vi "Handle.vi"(10 "log record":T1 {"timestamp" format="%<%x %.3X>T"}, 11 "logger in":refnum<class "Logger.lvclass">) -> (3 "logger out":refnum<class "Logger.lvclass">)   [LabVIEW 2018, in "GLog.lvlib" / "Logger.lvclass"]
uses:
  Logger.lvclass
  Log Record.ctl
  Internal Log Levels.ctl
  Logger.lvclass/Logger.ctl
  Failure Popup.vi
  <vilib>/ErrorRing/Error Ring.xnode
  extension/formatting_handler_interface/Formatting Handler.lvclass
  GLog.lvlib
panel:
  # "Connector Pane"
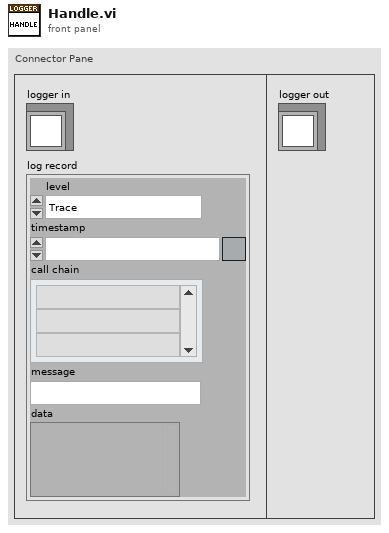
[diagram p1: front panel]
types:
  T1 = typedef "GLog.lvlib/Log Record.ctl" = cluster{"level":T2, "timestamp":timestamp, "call chain":string[], "message":string, "data":variant}
  T2 = typedef "GLog.lvlib/Internal Log Levels.ctl" = enum16{"Trace", "Debug", "Info", "Warning", "Error", "Critical", "Internal"}
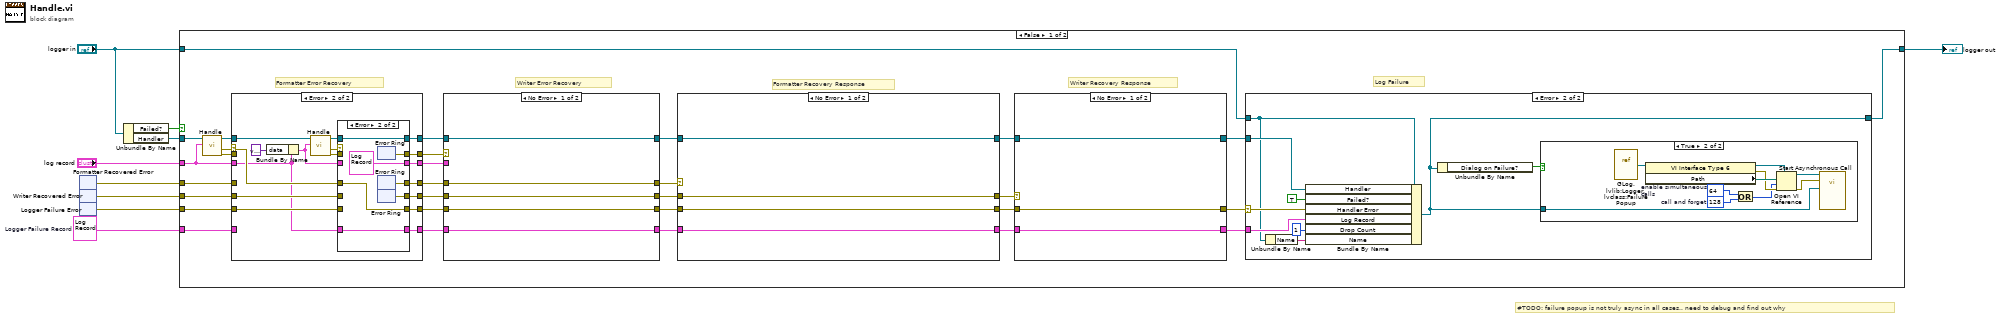
[diagram p0: block diagram]
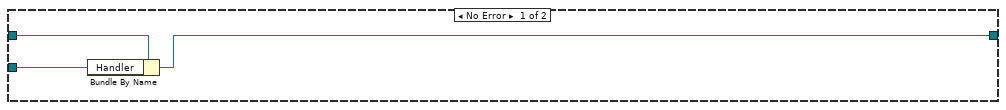
[diagram p2: hidden frame]
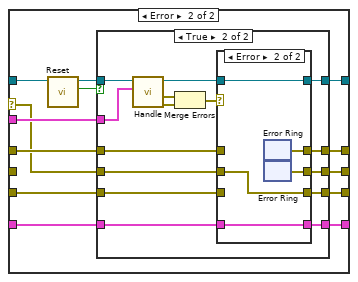
[diagram p6: hidden frame]
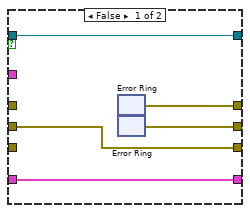
[diagram p7: hidden frame]
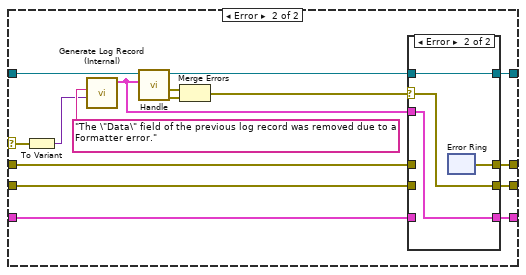
[diagram p9: hidden frame]
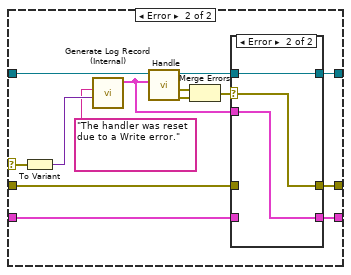
[diagram p11: hidden frame]
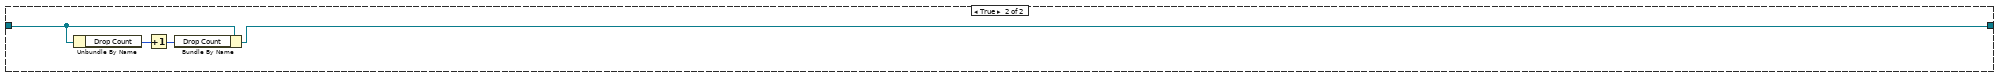
[diagram p13: hidden frame]
diagram:
  w9 = T1 {"level"=enum."Trace", "timestamp"=timestamp(0 s since 1904-01-01), "call chain"=[], "message"="", "data"=variant}  # Logger Failure Record
  # "#TODO: failure popup is not truly async in all cases.. need to debug and find out why"
  n1 = xnode "Formatter Recovered Error"() -> ("error out"=w6:errorcluster)
  n2 = xnode "Writer Recovered Error"() -> ("error out"=w7:errorcluster)
  n3 = xnode "Logger Failure Error"() -> ("error out"=w8:errorcluster)
  n4 = Unbundle By Name("logger in") -> ("Failed?"=w1:bool, "Handler"=w5:refnum<class "Formatting Handler.lvclass">)
  n5 = case shown="False" w1 {
    tunnel: w9 -> [w38 _]
    tunnel: w8 -> [w33 _]
    tunnel: w7 -> [w32 _]
    tunnel: w6 -> [w30 _]
    tunnel: w5 -> [w15 _]
    tunnel: "log record" -> [w13 _]
    tunnel: "logger in" -> [w11 w206]
    tunnel: [w10 w205] -> w2
    frame False {
      # "Log Failure"
      # "Writer Recovery Response"
      # "Formatter Recovery Response"
      # "Writer Error Recovery"
      # "Formatter Error Recovery"
      n6 = call-dynamic "Handle.vi"("log record"=w13, "handler in"=w15) -> ("writer error"=w16:errorcluster, "formatter error"=w12:errorcluster, "handler out"=w14:refnum<class "Formatting Handler.lvclass">)  [unwired: 7 in]
      n7 = case shown="Error" w12 {
        selector: w12 -> [_ w70]
        tunnel: w13 -> [w62 w68]
        tunnel: w14 -> [w63 w83]
        tunnel: w16 -> [w67 _]
        tunnel: [w67 w80] -> w17
        tunnel: [w66 w79] -> w18
        tunnel: [w64 w77] -> w19
        tunnel: w30 -> [w66 _]
        tunnel: w33 -> [w64 w78]
        tunnel: [w65 w76] -> w24
        tunnel: w32 -> [w65 w75]
        tunnel: [w63 w74] -> w27
        tunnel: [w62 w71] -> w28
        tunnel: [w62 w69] -> w37
        tunnel: w38 -> [_ _]
        frame No Error {
        }
        frame Error {
          n8 = Bundle By Name(cluster=w68, "data"=variant) -> (w72:T1)
          n9 = call-dynamic "Handle.vi"("log record"=w72, "handler in"=w83) -> ("writer error"=w81:errorcluster, "formatter error"=w82:errorcluster, "handler out"=w73:refnum<class "Formatting Handler.lvclass">)  [unwired: 7 in]
          n10 = case shown="Error" w82 {
            tunnel: w81 -> [w90 _]
            tunnel: [w90 w97] -> w80
            tunnel: [w86 w94] -> w79
            tunnel: [w89 w92] -> w77
            tunnel: w70 -> [w86 w92]
            tunnel: w78 -> [w89 _]
            tunnel: [w88 w93] -> w76
            tunnel: w75 -> [w88 _]
            tunnel: [w87 w96] -> w74
            tunnel: w73 -> [w87 w96]
            tunnel: [w85 T1 {"level"=enum."Trace", "timestamp"=timestamp(0 s since 1904-01-01), "call chain"=[], "message"="", "data"=variant} ("log record")] -> w71
            tunnel: w72 -> [w85 _]
            tunnel: [w85 w91] -> w69
            tunnel: w68 -> [_ w91]
            frame No Error {
            }
            frame Error {
              n11 = xnode "Error Ring"() -> ("error out"=w97:errorcluster)
              n12 = xnode "Error Ring"() -> ("error out"=w94:errorcluster)
              n13 = xnode "Error Ring"() -> ("error out"=w93:errorcluster)
            }
          }
        }
      }
      n14 = case shown="No Error" w17 {
        selector: w17 -> [_ w108]
        tunnel: w18 -> [w105 w113]
        tunnel: w19 -> [w104 w111]
        tunnel: [w105 w114] -> w20
        tunnel: [w104 w109] -> w23
        tunnel: [w103 w112] -> w26
        tunnel: w24 -> [w103 _]
        tunnel: w27 -> [w102 w118]
        tunnel: w28 -> [_ w115]
        tunnel: [w102 w110] -> w29
        tunnel: [w101 w107] -> w36
        tunnel: w37 -> [w101 w106]
        frame No Error {
        }
        frame Error {
          n15 = call-dynamic "Reset.vi"("handler in"=w118) -> ("successful?"=w116:bool, "handler out"=w117:refnum<class "Formatting Handler.lvclass">)  [unwired: 9 in]
          n16 = case shown="True" w116 {
            tunnel: w117 -> [w123 w140]
            tunnel: w115 -> [_ w136]
            tunnel: [w122 w135] -> w114
            tunnel: w113 -> [_ w134]
            tunnel: [w121 w133] -> w112
            tunnel: w108 -> [w120 w132]
            tunnel: w111 -> [_ w131]
            tunnel: [w123 w130] -> w110
            tunnel: [w120 w128] -> w109
            tunnel: [w119 w127] -> w107
            tunnel: w106 -> [w119 w126]
            frame False {
              n17 = xnode "Error Ring"() -> ("error out"=w122:errorcluster)
              n18 = xnode "Error Ring"() -> ("error out"=w121:errorcluster)
            }
            frame True {
              n19 = call-dynamic "Handle.vi"("log record"=w136, "handler in"=w140) -> ("writer error"=w138:errorcluster, "formatter error"=w139:errorcluster, "handler out"=w129:refnum<class "Formatting Handler.lvclass">)  [unwired: 7 in]
              n20 = Merge Errors(w139, w138) -> (w137:errorcluster)
              n21 = case shown="Error" w137 {
                tunnel: [w145 w149] -> w135
                tunnel: w134 -> [w145 _]
                tunnel: [w142 w148] -> w133
                tunnel: w132 -> [w142 w147]
                tunnel: w131 -> [w143 _]
                tunnel: [w144 w150] -> w130
                tunnel: w129 -> [w144 w150]
                tunnel: [w143 w147] -> w128
                tunnel: [w141 w146] -> w127
                tunnel: w126 -> [w141 w146]
                frame No Error {
                }
                frame Error {
                  n22 = xnode "Error Ring"() -> ("error out"=w149:errorcluster)
                  n23 = xnode "Error Ring"() -> ("error out"=w148:errorcluster)
                }
              }
            }
          }
        }
      }
      n24 = case shown="No Error" w20 {
        selector: w20 -> [_ w171]
        tunnel: [w156 w160] -> w22
        tunnel: w23 -> [w156 w164]
        tunnel: [w155 w161] -> w25
        tunnel: w26 -> [w155 w169]
        tunnel: w29 -> [w154 w172]
        tunnel: [w154 w162] -> w31
        tunnel: [w153 w159] -> w35
        tunnel: w36 -> [w153 w158]
        frame No Error {
        }
        frame Error {
          n25 = To Variant(anything=w171) -> (Variant=w163:variant)
          n26 = call "Generate Log Record (Internal).vi"("data (null)"=w163, "message (\"\")"="The \"Data\" field of the previous log record was removed due to a Formatter error." ("message (\"\")")) -> ("log record"=w157:T1)  [unwired: 9 in]
          n27 = call-dynamic "Handle.vi"("log record"=w157, "handler in"=w172) -> ("writer error"=w167:errorcluster, "formatter error"=w168:errorcluster, "handler out"=w165:refnum<class "Formatting Handler.lvclass">)  [unwired: 7 in]
          n28 = Merge Errors(w168, w167) -> (w166:errorcluster)
          n29 = case shown="Error" w166 {
            selector: w166 -> [_ w178]
            tunnel: w169 -> [w175 _]
            tunnel: w165 -> [w176 w180]
            tunnel: w164 -> [w174 _]
            tunnel: [w176 w180] -> w162
            tunnel: [w175 w179] -> w161
            tunnel: [w174 w178] -> w160
            tunnel: [w173 w177] -> w159
            tunnel: w158 -> [w173 _]
            tunnel: w157 -> [_ w177]
            frame No Error {
            }
            frame Error {
              n30 = xnode "Error Ring"() -> ("error out"=w179:errorcluster)
            }
          }
        }
      }
      n31 = case shown="No Error" w25 {
        selector: w25 -> [_ w192]
        tunnel: [w184 w189] -> w21
        tunnel: w22 -> [w184 w191]
        tunnel: w31 -> [w182 w193]
        tunnel: [w183 w188] -> w34
        tunnel: w35 -> [w183 w187]
        tunnel: [w182 w185] -> w39
        frame No Error {
        }
        frame Error {
          n32 = To Variant(anything=w192) -> (Variant=w194:variant)
          n33 = call "Generate Log Record (Internal).vi"("data (null)"=w194, "message (\"\")"="The handler was reset due to a Write error." ("message (\"\")")) -> ("log record"=w186:T1)  [unwired: 9 in]
          n34 = call-dynamic "Handle.vi"("log record"=w186, "handler in"=w193) -> ("writer error"=w197:errorcluster, "formatter error"=w198:errorcluster, "handler out"=w195:refnum<class "Formatting Handler.lvclass">)  [unwired: 7 in]
          n35 = Merge Errors(w198, w197) -> (w196:errorcluster)
          n36 = case shown="Error" w196 {
            selector: w196 -> [_ w203]
            tunnel: w195 -> [w201 w204]
            tunnel: w191 -> [w200 _]
            tunnel: [w201 w204] -> w185
            tunnel: [w200 w203] -> w189
            tunnel: [w199 w202] -> w188
            tunnel: w187 -> [w199 _]
            tunnel: w186 -> [_ w202]
            frame No Error {
            }
            frame Error {
            }
          }
        }
      }
      n37 = case shown="Error" w21 {
        selector: w21 -> [_ w49]
        tunnel: w11 -> [w42 w44]
        tunnel: w34 -> [_ w50]
        tunnel: [w41 w46] -> w10
        tunnel: w39 -> [w40 w47]
        frame No Error {
          n38 = Bundle By Name(cluster=w42, "Handler"=w40) -> (w41:refnum<class "Logger.lvclass">)
        }
        frame Error {
          n39 = Unbundle By Name(w44) -> ("Name"=w43:string)
          n40 = Bundle By Name(cluster=w44, "Handler"=w47, "Failed?"=TRUE, "Handler Error"=w49, "Log Record"=w50, "Drop Count"=u32 1 ("Fail Info.Drop Count"), "Name"=w43) -> (w46:refnum<class "Logger.lvclass">)
          n41 = Unbundle By Name(w46) -> ("Dialog on Failure?"=w45:bool)
          n42 = case shown="True" w45 {
            tunnel: w46 -> [_ w55]
            frame False {
            }
            frame True {
              w53 = 128  # call and forget
              w54 = 64  # enable simultaneous calls
              n43 = vi-ref "GLog.lvlib:Logger.lvclass:Failure Popup.vi"() -> (w61:refnum<vi>)
              n44 = property class="VI Interface Type 6"(reference=w61) -> (reference out=w58:refnum<vi>, error out=w59:errorcluster, "Path"=w60:path)  [unwired: 1 in]
              n45 = Compound Arithmetic op=OR(w54, w53) -> (w52:i32)
              n46 = Open VI Reference(type specifier VI Refnum (for type only)=w58, vi path=w60, options=w52, error in (no error)=w59) -> (vi reference=w56:refnum<vi>, error out=w57:errorcluster)  [unwired: 2 in]
              n47 = call-by-ref "Start Asynchronous Call"(reference=w56, error in=w57, "Logger in"=w55) -> ()  [unwired: 11 in, 2 out]
            }
          }
        }
      }
    }
    frame True {
      n48 = Unbundle By Name(w206) -> ("Drop Count"=w208:u32)
      n49 = Increment(x=w208) -> (x+1=w207:u32)
      n50 = Bundle By Name(cluster=w206, "Drop Count"=w207) -> (w205:refnum<class "Logger.lvclass">)
    }
  }
  "logger out" <- w2
